vi "打包属性.vi"(4 "方向":string, 6 "功能":string, 8 "样品标记":string, 10 "错误输入（无错误）":errorcluster) -> (2 "错误输出":errorcluster, 3 "数据属性":T1)   [LabVIEW 2021]
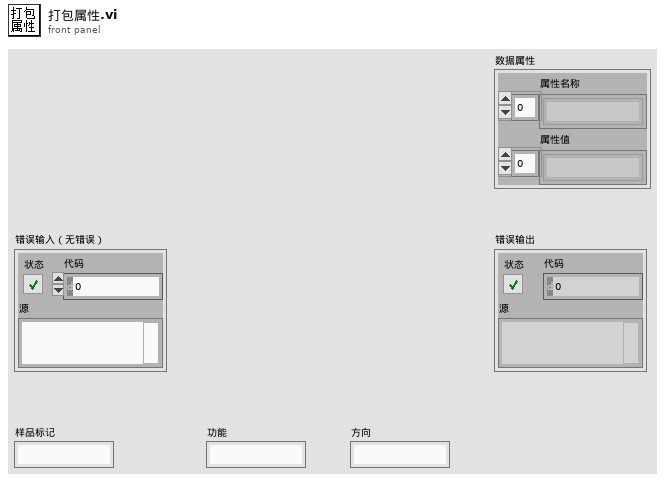
[diagram p1: front panel]
types:
  T1 = typedef "数据属性.ctl" = cluster{"属性名称":string[], "属性值":string[]}
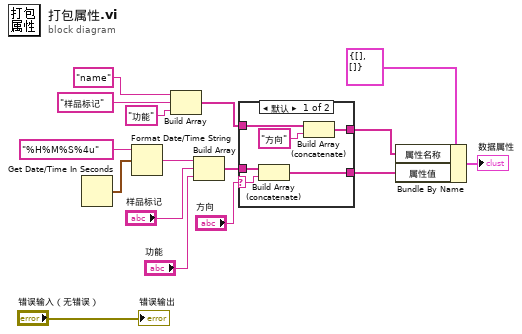
[diagram p0: block diagram]
diagram:
  n1 = Get Date/Time In Seconds() -> (seconds since 1Jan1904=w14:timestamp)
  n2 = Format Date/Time String(time format string (%c)="%H%M%S%4u" ("时间格式字符串(%c)"), seconds (now)=w14) -> (date/time string=w13:string)  [unwired: 1 in]
  n3 = Build Array("name" ("元素"), "样品标记" ("元素"), "功能" ("元素")) -> (w9:string[])
  n4 = Build Array(w13, "样品标记", "功能") -> (w8:string[])
  n5 = case shown="默认" "方向" {
    selector: "方向" -> [w17 _]
    tunnel: w9 -> [w22 w24]
    tunnel: w8 -> [w20 w23]
    tunnel: [w19 w24] -> w5
    tunnel: [w18 w23] -> w4
    frame Default {
      n6 = Build Array (concatenate)(w20, w17) -> (w18:string[])
      n7 = Build Array (concatenate)(w22, "方向" ("元素")) -> (w19:string[])
    }
    frame "" {
    }
  }
  n8 = Bundle By Name(cluster=T1 {"属性名称"=[], "属性值"=[]} ("数据属性"), "属性名称"=w5, "属性值"=w4) -> (→"数据属性":T1)
  "错误输出" <- "错误输入（无错误）"
